vi "Get Server State Ref.vi"(11 "Template Server in":refnum<class "TestServer.lvclass">) -> (2 "Server State Ref":refnum<data-value>, 3 "Template Server out":refnum<class "TestServer.lvclass">)   [LabVIEW 2019, in "TestServer.lvlib" / "TestServer.lvclass"]
uses:
  TestServer.lvclass
  typeDefs/Server State Data.ctl
  TestServer.lvclass/TestServer.ctl
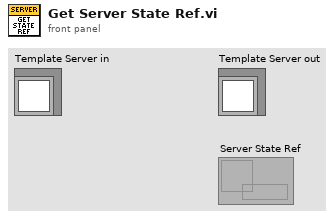
[diagram p1: front panel]
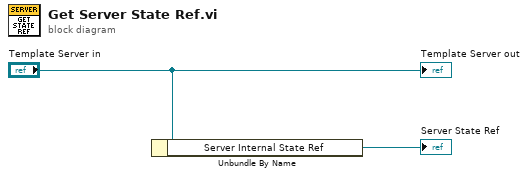
[diagram p0: block diagram]
diagram:
  n1 = Unbundle By Name("Template Server in") -> ("Server Internal State Ref"=→"Server State Ref":refnum<data-value>)
  "Template Server out" <- "Template Server in"
